vi "MB_relay_01_encode.vi"(8 "error in (no error)":errorcluster, 10 "eMic1-6":bool[](array[boolean])=[FALSE, FALSE, FALSE, FALSE, FALSE, FALSE], 11 "Mem_mapping in":u16[](array[numeric])) -> (0 "error out":errorcluster, 3 "MemMapping Out":u16[](array[numeric]))   [LabVIEW 2018, in "MB Relay.lvlib"]
uses:
  MB Relay.lvlib
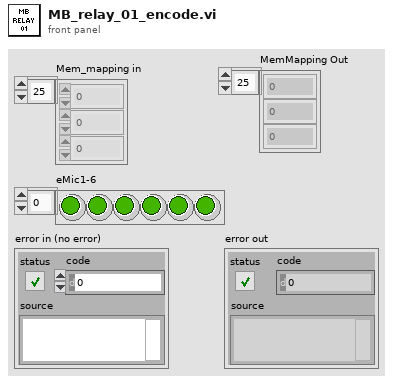
[diagram p1: front panel]
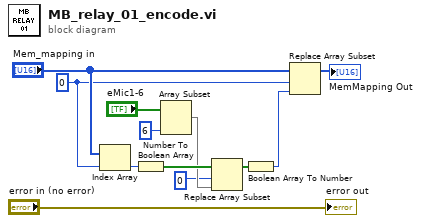
[diagram p0: block diagram]
diagram:
  w9 = 0 ("index")
  n1 = Index Array(array="Mem_mapping in", index=w9) -> (element=w8:u16)
  n2 = Number To Boolean Array(number=w8) -> (Boolean array=w5:bool[])
  n3 = Array Subset(array="eMic1-6", length=6) -> (w4:bool[])  [unwired: 1 in]
  n4 = Replace Array Subset(array=w5, new element=w4, index=0) -> (w2:bool[])
  n5 = Boolean Array To Number(Boolean array=w2) -> (number=w1:u16)
  n6 = Replace Array Subset(array="Mem_mapping in", new element=w1, index=w9) -> (→"MemMapping Out":u16[])
  "error out" <- "error in (no error)"
